vi "Add Process to Map.vi"(8 "error in (no error)":errorcluster, 10 "Process Out":refnum<class "Process.lvclass">, 11 "Application in":refnum<class "Application.lvclass">) -> (0 "error out":errorcluster, 3 "Application out":refnum<class "Application.lvclass">)   [LabVIEW 2020, in "Application.lvclass"]
uses:
  Application.lvclass
  Process/Process.lvclass
  Application.lvclass/Application.ctl
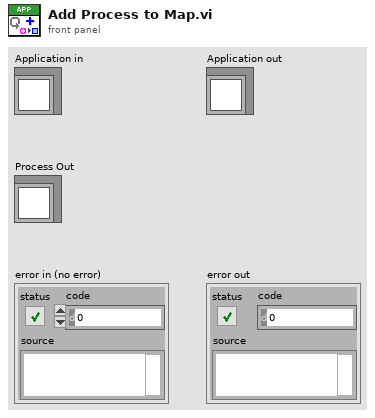
[diagram p1: front panel]
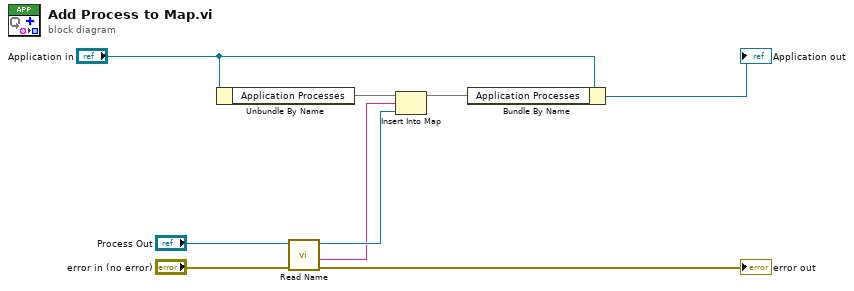
[diagram p0: block diagram]
diagram:
  n1 = Unbundle By Name("Application in") -> ("Application Processes"=w2:map{string, refnum<class "Process.lvclass">})
  n2 = call-dynamic "Read Name.vi"("error in (no error)"="error in (no error)", "Process In"="Process Out") -> ("error out"=→"error out":errorcluster, "Name"=w1:string, "Process Out"=w4:refnum<class "Process.lvclass">)  [unwired: 6 in, 1 out]
  n3 = Insert Into Map(map in=w2, key=w1, value=w4) -> (map out=w3:map{string, refnum<class "Process.lvclass">})  [unwired: 2 out]
  n4 = Bundle By Name(cluster="Application in", "Application Processes"=w3) -> (→"Application out":refnum<class "Application.lvclass">)
